vi "PRACTICA 3 CONTROL DE NIVEL DE TANQUE.vi"() -> ()   [LabVIEW 2017]
panel:
  out "TANQUE":dbl(slide) scale=0.0..100.0
  out "BOMBA 2":bool
  out "BOMBA 1":bool
  out "LIMITE MEDIO":dbl
  in  "LIMITE INFERIOR":dbl
  in  "LIMITE SUPERIOR":dbl
  in  "SENSOR":dbl(slide) scale=0.0..100.0
  # "PRACTICA 3 CONTROL DE NIVEL DE TANQUE"
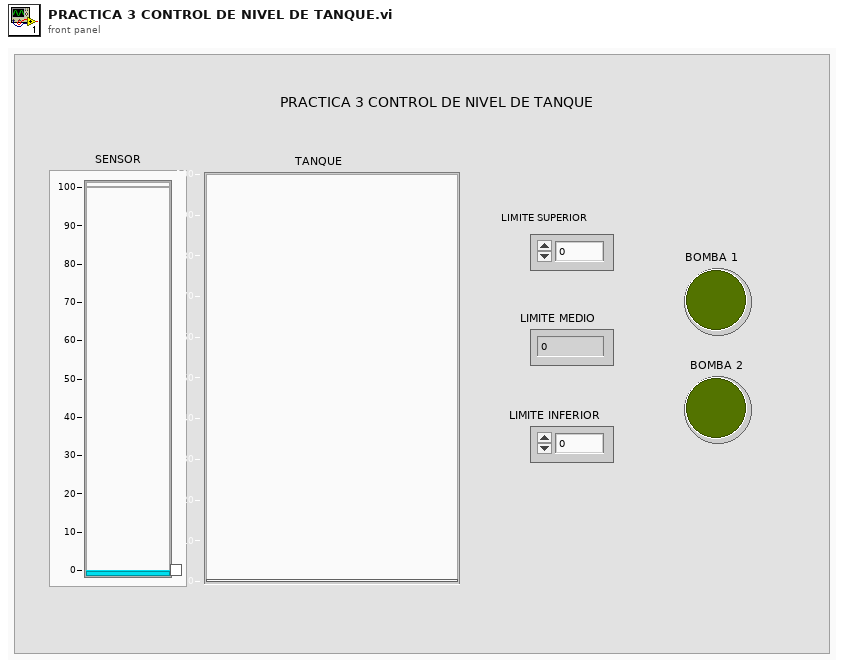
[diagram p1: front panel]
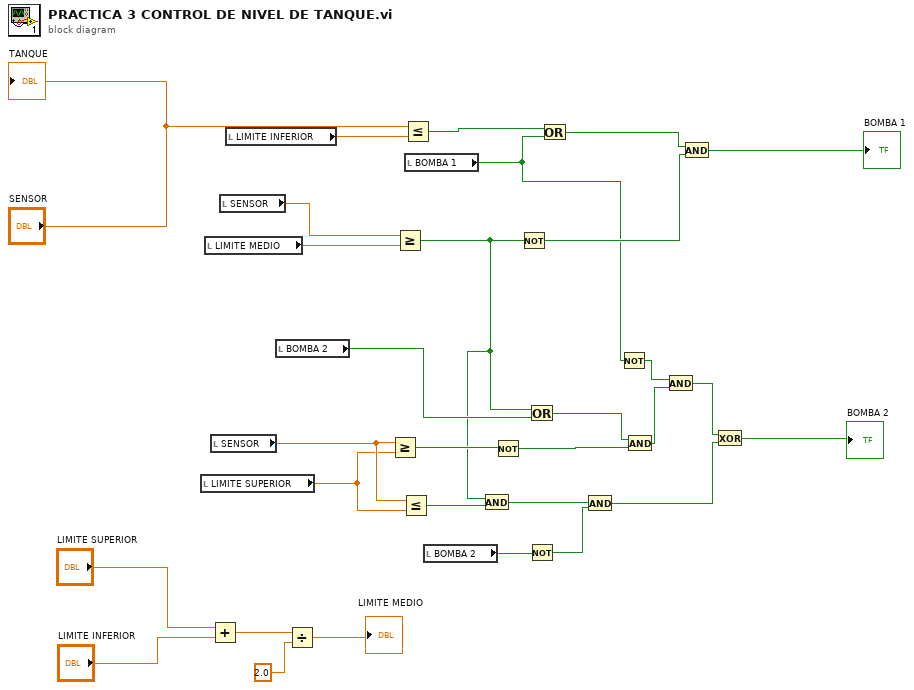
[diagram p0: block diagram]
diagram:
  n1 = local read "LIMITE SUPERIOR"() -> (w10:dbl)
  n2 = local read "LIMITE MEDIO"() -> (w24:dbl)
  n3 = Add(x="LIMITE SUPERIOR", y="LIMITE INFERIOR") -> (x+y=w28:dbl)
  n4 = local read "SENSOR"() -> (w11:dbl)
  n5 = local read "SENSOR"() -> (w23:dbl)
  n6 = local read "LIMITE INFERIOR"() -> (w19:dbl)
  n7 = local read "BOMBA 2"() -> (w18:bool)
  n8 = Divide(x=w28, y=2.0) -> (x/y=→"LIMITE MEDIO":dbl)
  n9 = Greater Or Equal?(x=w11, y=w10) -> (x >= y?=w17:bool)
  n10 = Greater Or Equal?(x=w23, y=w24) -> (x >= y?=w9:bool)
  n11 = Less Or Equal?(x=w11, y=w10) -> (x <= y?=w8:bool)
  n12 = Less Or Equal?(x="SENSOR", y=w19) -> (x <= y?=w21:bool)
  n13 = local read "BOMBA 1"() -> (w14:bool)
  n14 = local read "BOMBA 2"() -> (w5:bool)
  n15 = And(x=w9, y=w8) -> (x .and. y?=w6:bool)
  n16 = Not(x=w17) -> (.not. x?=w15:bool)
  n17 = Not(x=w9) -> (.not. x?=w22:bool)
  n18 = Or(x=w9, y=w18) -> (x .or. y?=w16:bool)
  n19 = Not(x=w5) -> (.not. x?=w4:bool)
  n20 = Or(x=w21, y=w14) -> (x .or. y?=w25:bool)
  n21 = And(x=w6, y=w4) -> (x .and. y?=w3:bool)
  n22 = Not(x=w14) -> (.not. x?=w13:bool)
  n23 = And(x=w16, y=w15) -> (x .and. y?=w12:bool)
  n24 = And(x=w13, y=w12) -> (x .and. y?=w7:bool)
  n25 = And(x=w25, y=w22) -> (x .and. y?=→"BOMBA 1":bool)
  n26 = Exclusive Or(1:w3, 2:w7) -> (0:→"BOMBA 2":bool)
  "TANQUE" <- "SENSOR"
